vi "csv (1).vi"() -> ()   [LabVIEW 2016]
uses:
  <vilib>/Analysis/1siggen.llb/Ramp Pattern by Samples.vi
  <vilib>/Utility/file.llb/Read Delimited Spreadsheet (string).vi
  <vilib>/Analysis/NI_AALPro.lvlib
  <vilib>/gmath/NI_Gmath.lvlib
  <vilib>/Analysis/NI_AALBase.lvlib
panel:
  out "RRI":T1(graph)
  out "R-peak":cluster{i32[], dbl[]}(graph)={[346, 950, 1546, 2132, 2718, 3309, 3910, 4510, 5105, 5704, 6311, 6938, 7590, 8233, 8869, 9512, 10151, 10801, 11427, 12040, 12652, 13257, 13861, 14460, 15053, 15646, 16242, 16848, 17474, 18103, 18729, 18731, 19369, 20017, 20672, 21303, 21919, 22529, 23138, 23743, 24344, 24943, 25542, 26144, 26742, 27352, 27968, 28566, 29171, 29785], [-0.338281, -0.348693, -0.355333, -0.340119, -0.357687, -0.34173, -0.34937, -0.339925, -0.324775, -0.298922, -0.326902, -0.326, -0.313106, -0.324581, -0.314137, -0.331383, -0.336186, -0.333833, -0.352336, -0.330416, -0.335025, -0.340795, -0.349596, -0.337411, -0.342536, -0.325742, -0.34144, -0.343374, -0.323775, -0.32629, -0.340473, -0.313782, -0.345566, -0.336379, -0.324162, -0.328997, -0.326548, -0.340183, -0.350015, -0.338765, -0.3436, -0.324871, -0.337379, -0.32774, -0.335541, -0.322583, -0.315201, -0.332672, -0.316813, -0.321906]}
  out "驗證找出的peak對不對":cluster{i32[], "Waveform Graph 3":dbl[]}[](graph)=[{array[30000 elements], "Waveform Graph 3"=array[30000 elements]}, {[346, 950, 1546, 2132, 2718, 3309, 3910, 4510, 5105, 5704, 6311, 6938, 7590, 8233, 8869, 9512, 10151, 10801, 11427, 12040, 12652, 13257, 13861, 14460, 15053, 15646, 16242, 16848, 17474, 18103, 18729, 18731, 19369, 20017, 20672, 21303, 21919, 22529, 23138, 23743, 24344, 24943, 25542, 26144, 26742, 27352, 27968, 28566, 29171, 29785], "Waveform Graph 3"=[-0.338281, -0.348693, -0.355333, -0.340119, -0.357687, -0.34173, -0.34937, -0.339925, -0.324775, -0.298922, -0.326902, -0.326, -0.313106, -0.324581, -0.314137, -0.331383, -0.336186, -0.333833, -0.352336, -0.330416, -0.335025, -0.340795, -0.349596, -0.337411, -0.342536, -0.325742, -0.34144, -0.343374, -0.323775, -0.32629, -0.340473, -0.313782, -0.345566, -0.336379, -0.324162, -0.328997, -0.326548, -0.340183, -0.350015, -0.338765, -0.3436, -0.324871, -0.337379, -0.32774, -0.335541, -0.322583, -0.315201, -0.332672, -0.316813, -0.321906]}]
  out "PS?":T2(graph)
  out "ORIGIN":cluster{dbl[], dbl[]}(graph)
  out "Data Dsiplay 3":dbl[](array[numeric])
  out "Data Dsiplay 2":dbl[][](array[numeric])
  in  "CSV FILE PATH":path
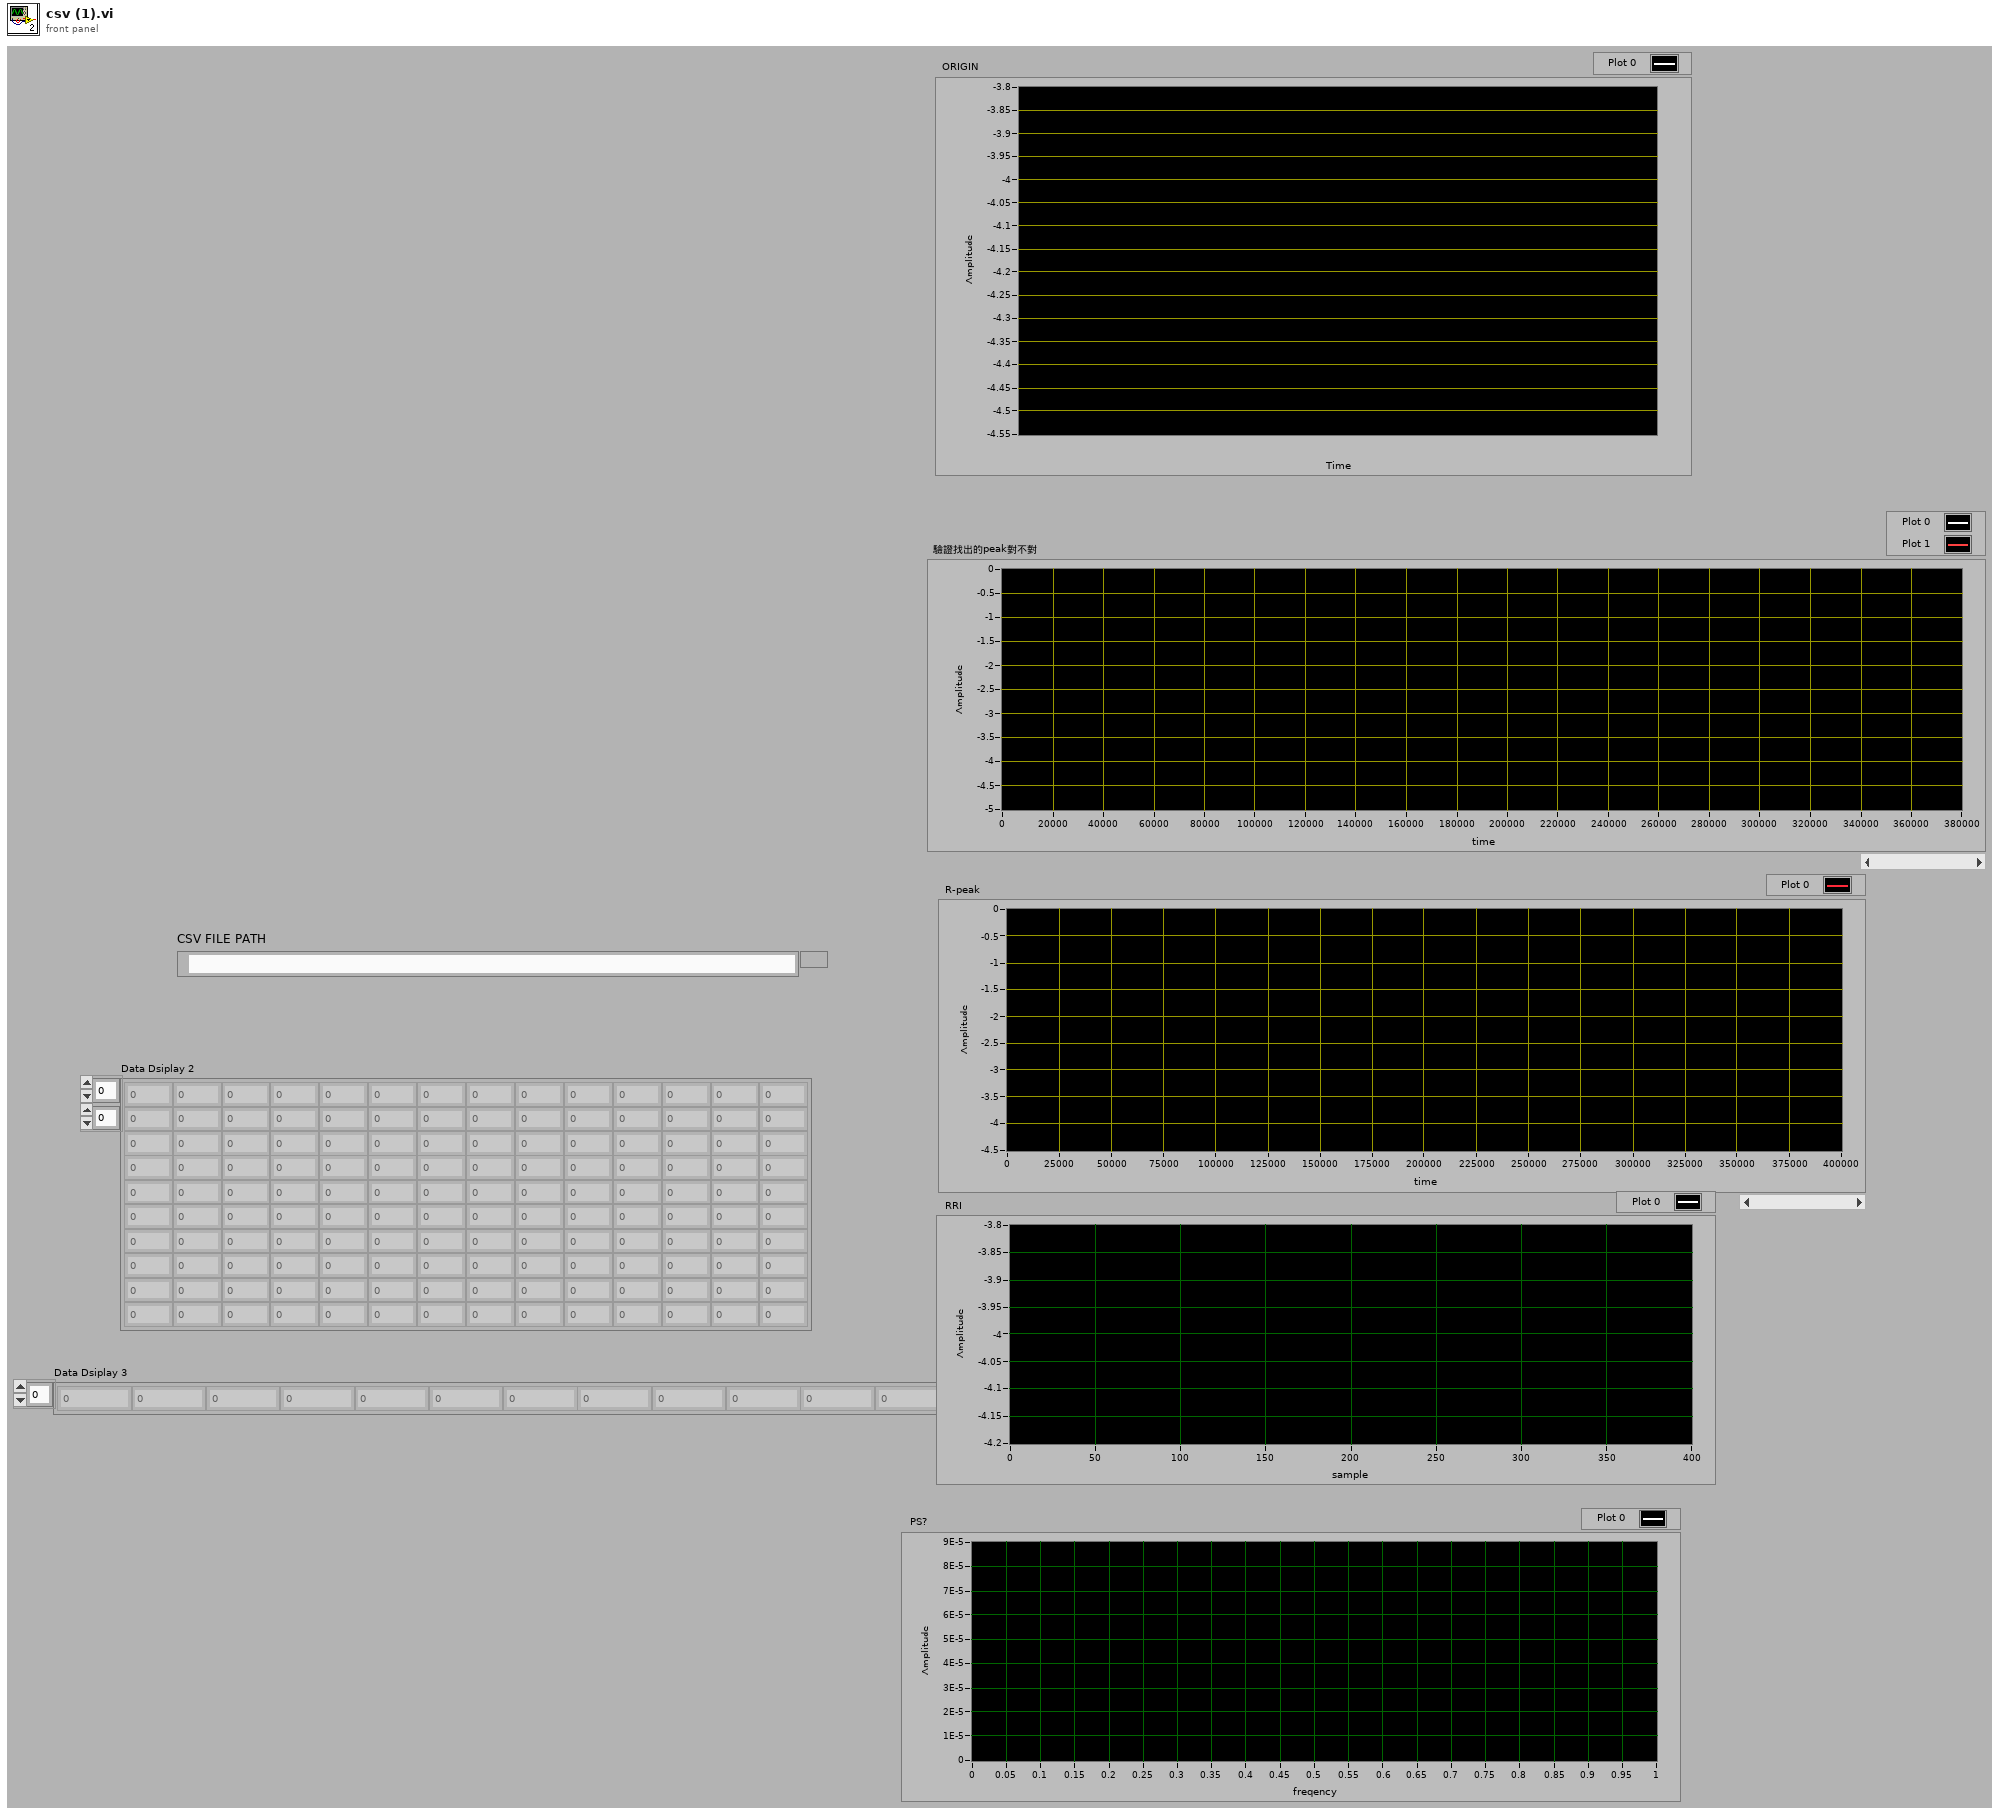
[diagram p1: front panel]
types:
  T1 = cluster{i32, "df":dbl, "Power Spectrum (V^2 rms)":dbl[]}
  T2 = cluster{i32, dbl, "Power Spectrum (V^2 rms)":dbl[]}
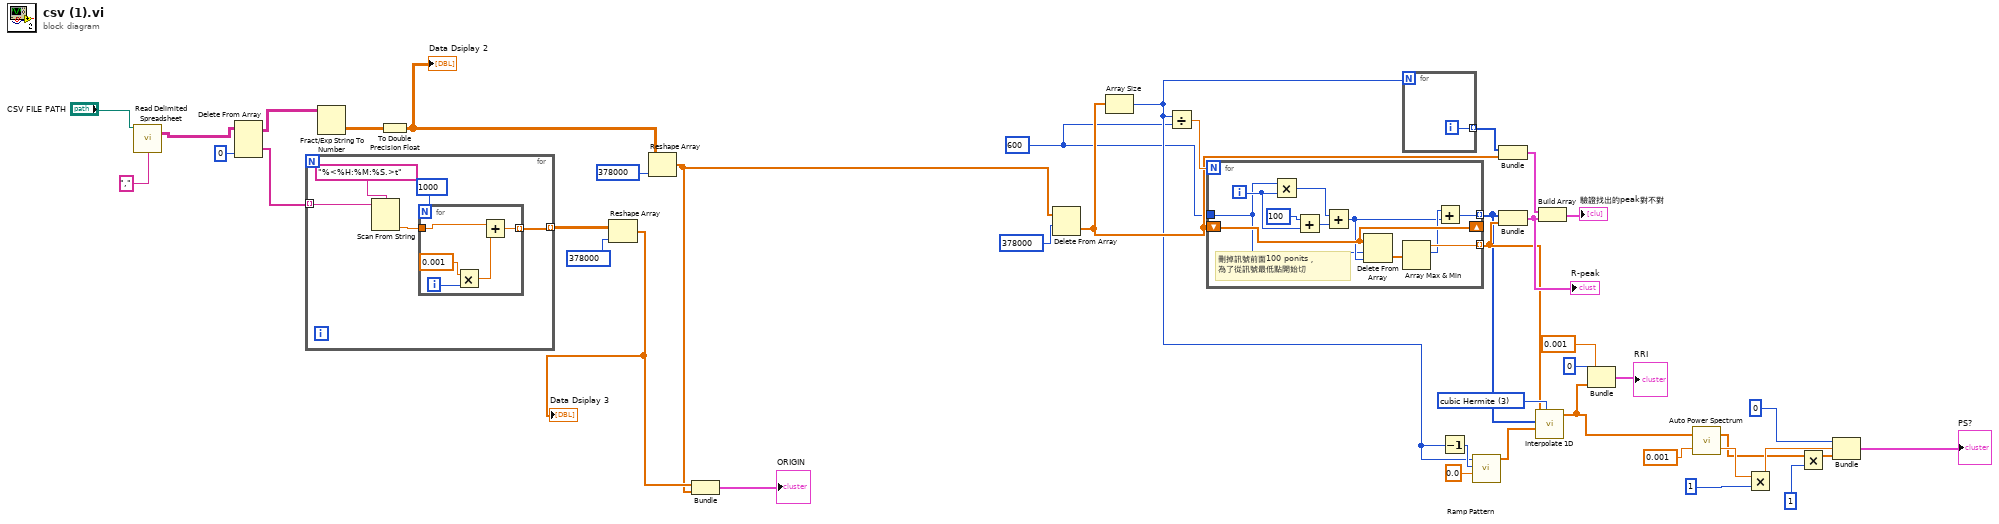
[diagram p0: block diagram]
diagram:
  w22 = 3 items=["nearest", "linear", "spline", "cubic Hermite", "Lagrange"] ("method")
  w16 = 600 ("y")
  n1 = call-poly <vilib>:"Read Delimited Spreadsheet.vi"("file path (dialog if empty)"="CSV FILE PATH", "delimiter (\\t)"="," ("delimiter (\\t)")) -> ("all rows"=w30:string[][])  [unwired: 8 in, 5 out]
  n2 = Delete From Array(array=w30, index (col)=0 ("disabled index (col)")) -> (deleted portion=w37:string[], array with subset deleted=w38:string[][])  [unwired: 2 in]
  n3 = for {
    tunnel: w37 -> [w46] mode=indexing
    tunnel: [w43] -> w36 mode=indexing
    n4 = Scan From String(format string="%<%H:%M:%S.>t", input string=w46) -> (output 1=w45:dbl)  [unwired: 3 in, 3 out]
    n5 = for {
      N: 1000 -> [_]
      tunnel: w45 -> [w50]
      tunnel: [w48] -> w43 mode=indexing
      i -> [w51]
      n6 = Multiply(x=0.001, y=w51) -> (x*y=w49:dbl)
      n7 = Add(x=w50, y=w49) -> (x+y=w48:dbl)
    }
  }
  n8 = Fract/Exp String To Number(string=w38) -> (number=w39:dbl[][])  [unwired: 3 in, 1 out]
  n9 = To Double Precision Float(number=w39) -> (double precision float=w34:dbl[][])
  "Data Dsiplay 2" <- w34
  n10 = Reshape Array(w36, 378000 ("dimension size")) -> (w31:dbl[])
  "Data Dsiplay 3" <- w31
  n11 = Reshape Array(w34, 378000 ("dimension size")) -> (w17:dbl[])
  n12 = Bundle(w31, w17) -> (→"ORIGIN":cluster{dbl[], dbl[]})  [unwired: 1 in]
  n13 = Delete From Array(array=w17, length=378000) -> (deleted portion=w26:dbl[])  [unwired: 1 in, 1 out]
  n14 = Array Size(array=w26) -> (size(s)=w19:i32)
  n15 = Divide(x=w19, y=w16) -> (x/y=w28:dbl)
  n16 = for {
    N: w28 -> [_]
    shift-right: [w59] -> _
    shift-left: w26 -> [w59]
    tunnel: [w57] -> w15 mode=indexing
    tunnel: [w54] -> w11 mode=indexing
    tunnel: w16 -> [w53]
    i -> [w62]
    # "刪掉訊號前面100 ponits，\n為了從訊號最低點開始切"
    n17 = Multiply(x=w53, y=w62) -> (x*y=w61:i32)
    n18 = Add(x=100, y=w62) -> (x+y=w60:i32)
    n19 = Add(x=w61, y=w60) -> (x+y=w55:i32)
    n20 = Delete From Array(array=w59, length=w53, index=w55) -> (deleted portion=w58:dbl[])  [unwired: 1 out]
    n21 = Array Max & Min(array=w58) -> (max value=w57:dbl, max index (indices)=w56:i32)  [unwired: 2 out]
    n22 = Add(x=w56, y=w55) -> (x+y=w54:i32)
  }
  n23 = for {
    N: w19 -> [_]
    tunnel: [w64] -> w27 mode=indexing
    i -> [w64]
  }
  n24 = Decrement(x=w19) -> (x-1=w21:i32)
  n25 = call-poly <vilib>:"Ramp Pattern.vi"("start"=0.0, "end"=w21, "samples"=w19) -> ("Ramp Pattern"=w18:dbl[])  [unwired: 7 in, 1 out]
  n26 = Bundle(w27, w26) -> (w25:cluster{i32[], dbl[]})  [unwired: 1 in]
  n27 = Bundle(w11, w15) -> (w23:cluster{i32[], dbl[]})  [unwired: 1 in]
  "R-peak" <- w23
  n28 = call <vilib>:"Interpolate 1D.vi"("method"=w22, "xi"=w18, "X"=w11, "Y"=w15) -> ("yi"=w3:dbl[])  [unwired: 2 in, 5 out]
  n29 = Build Array(w25, w23) -> (→"驗證找出的peak對不對":cluster{i32[], dbl[]}[])
  n30 = Bundle(0, 0.001, "yi"=w3) -> (→"RRI":cluster{i32, dbl, "yi":dbl[]})  [unwired: 1 in]
  n31 = call <vilib>:"Auto Power Spectrum.vi"("dt"=0.001, "Signal (V)"=w3) -> ("df"=w12:dbl, "Power Spectrum (V^2 rms)"=w4:dbl[])
  n32 = Multiply(x=w12, y=1) -> (x*y=w10:dbl)
  n33 = Multiply(x=w4, y=1) -> (x*y=w2:dbl[])
  n34 = Bundle(0, w10, w2) -> (→"PS?":cluster{i32, dbl, dbl[]})  [unwired: 1 in]
